vi "XBox Controller.vi"() -> ()   [LabVIEW 2015]
uses:
  XBox-Button States.ctl
  Microsoft.Xna.Framework
  XBox-Globals.vi
panel:
  out "Connected?":bool
  out "Mouse Wheel":i32
  out "Right Trigger":dbl(slide) scale=0.0..1.0
  out "Left Trigger":dbl(slide) scale=0.0..1.0
  out "LeftX":dbl(slide) scale=-1.0..1.0
  out "LeftY":dbl(slide) scale=-1.0..1.0
  out "Left Stick":bool
  out "Left":bool
  out "Right":bool
  out "Down":bool
  out "Up":bool
  out "Right Stick":bool
  out "RightX":dbl(slide) scale=-1.0..1.0
  out "RightY":dbl(slide) scale=-1.0..1.0
  out "Back":bool
  out "Start":bool
  out "Big Button":bool
  out "Left":bool
  out "Right":bool
  out "X":bool
  out "A":bool
  out "B":bool
  out "Y":bool
  in  "Quit":bool
  in  "poll interval (ms)":u32=100
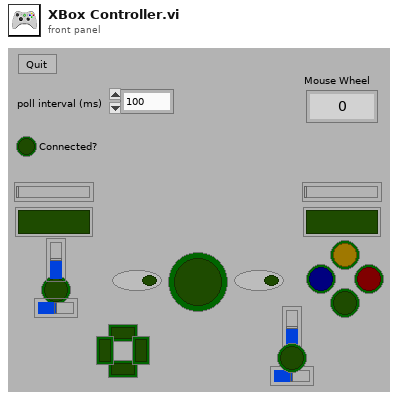
[diagram p1: front panel]
types:
  T1 = typedef "XBox-Button States.ctl" = cluster{"A":bool, "B":bool, "X":bool, "Y":bool, "Left":bool, "Right":bool, "Left Stick":bool, "Right Stick":bool, "Back":bool, "Start":bool, "DPad Down":bool, "DPad Up":bool, "DPad Left":bool, "DPad Right":bool}
  T2 = cluster{"Connected":refnum<user-event>, "A Button":refnum<user-event>, "B Button":refnum<user-event>, "X Button":refnum<user-event>, "Y Button":refnum<user-event>, "Left Button":refnum<user-event>, "Right Button":refnum<user-event>, "Left X":refnum<user-event>, "Left Y":refnum<user-event>, "Right X":refnum<user-event>, "Right Y":refnum<user-event>, "Right Trigger":refnum<user-event>, "Right Trigger":refnum<user-event>, "DPad Left":refnum<user-event>, "DPad Right":refnum<user-event>, "DPad Up":refnum<user-event>, "DPad Down":refnum<user-event>, "Mouse Wheel":refnum<user-event>, "Left Stick":refnum<user-event>, "Right Stick":refnum<user-event>, "Back":refnum<user-event>, "Start":refnum<user-event>, "Left XY":refnum<user-event>}
  T3 = typedef "XBox-Events Ref.ctl" = refnum<event-registration>
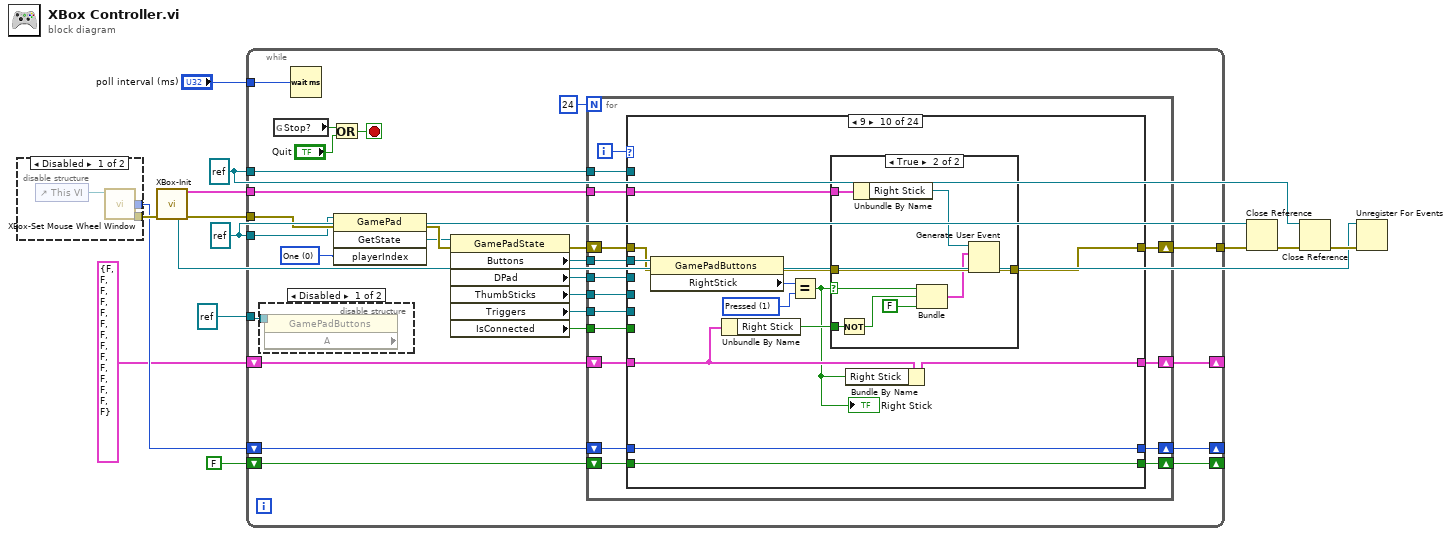
[diagram p0: block diagram]
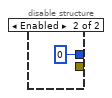
[diagram p2: hidden frame]
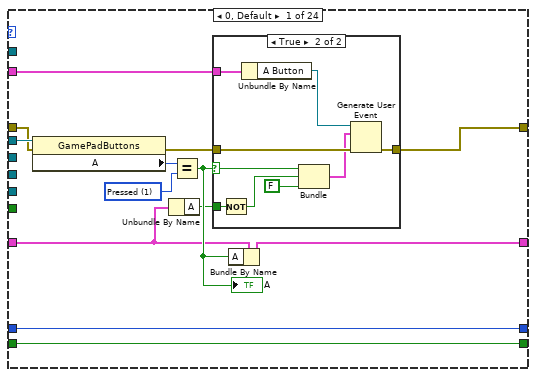
[diagram p4: hidden frame]
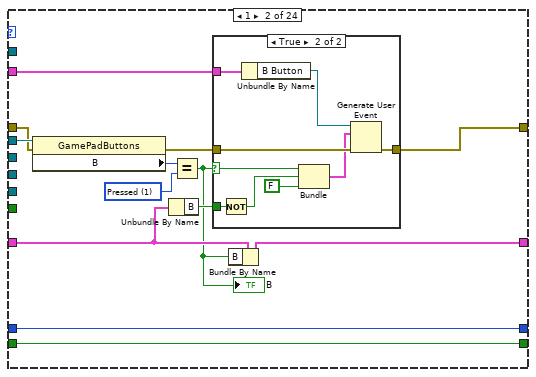
[diagram p6: hidden frame]
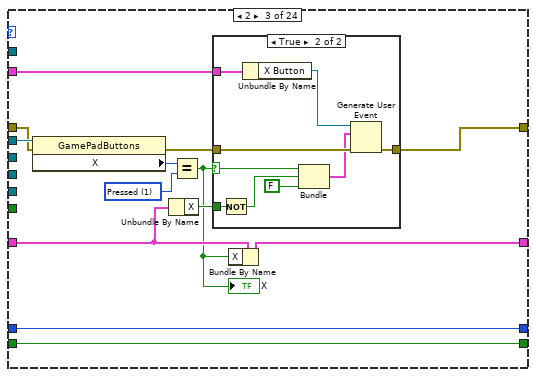
[diagram p8: hidden frame]
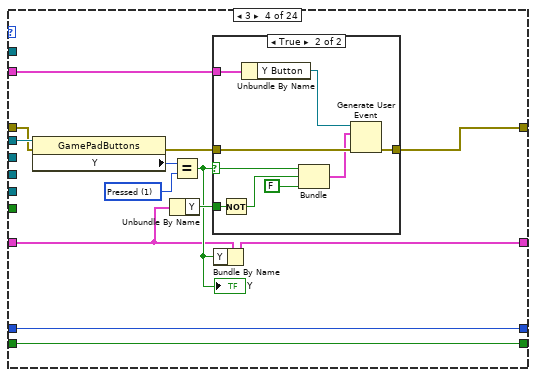
[diagram p10: hidden frame]
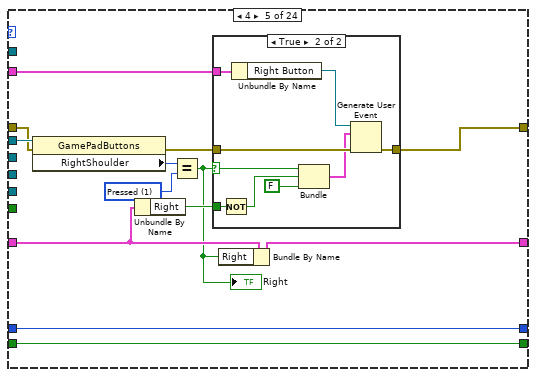
[diagram p12: hidden frame]
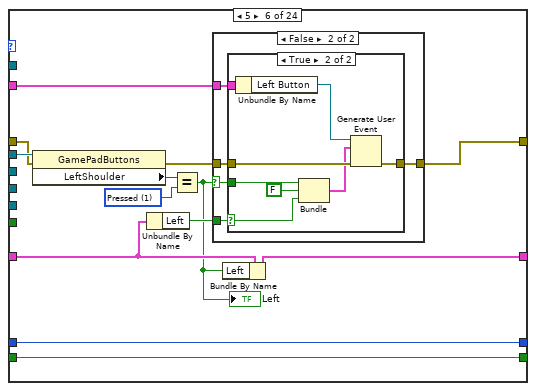
[diagram p14: hidden frame]
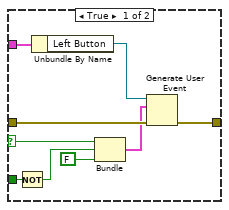
[diagram p15: hidden frame]
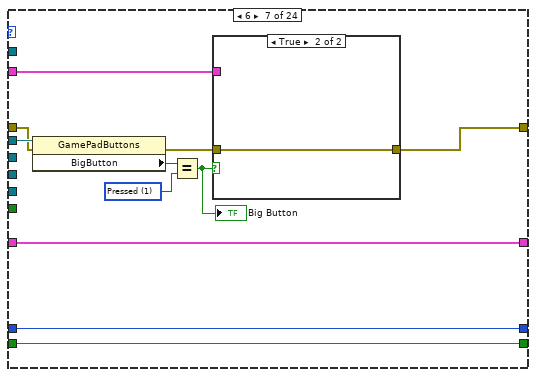
[diagram p17: hidden frame]
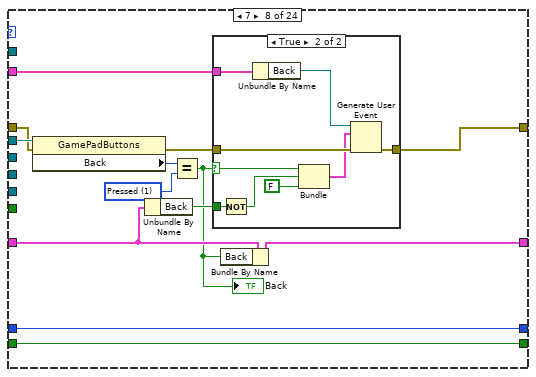
[diagram p19: hidden frame]
diagram:
  w5 = refnum<k24> refnum ("reference")
  w7 = refnum<k24> refnum ("reference")
  n1 = disable-structure shown="Disabled" {
    disable-tunnel: [w16 _] -> w11
    disable-tunnel: [w15 0 ("ScrollWheelValue")] -> w10
    frame Disabled {
      n2 = control-ref of="This VI"() -> (w17:refnum<vi>)
      n3 = call "XBox-Set Mouse Wheel Window.vi"("VI ref"=w17) -> ("ScrollWheelValue"=w15:i32, "error out"=w16:errorcluster)  [unwired: 13 in]
    }
    frame Enabled {
    }
  }
  n4 = call "XBox-Init.vi"("error in (no error)"=w11) -> ("XBox Events"=w12:T2, "Events Ref"=w3:T3, "error out"=w13:errorcluster)  [unwired: 12 in]
  n5 = while {
    tunnel: w12 -> [w39]
    tunnel: "poll interval (ms)" -> [w44]
    tunnel: w13 -> [w38]
    shift-right: [w28] -> _
    shift-left: w10 -> [w29]
    shift-right: [w26] -> _
    shift-left: FALSE -> [w27]
    tunnel: w7 -> [w20]
    tunnel: [w25] -> w8
    tunnel: w5 -> [w24]
    shift-right: [w22] -> _
    shift-left: T1 {"A"=FALSE, "B"=FALSE, "X"=FALSE, "Y"=FALSE, "Left"=FALSE, "Right"=FALSE, "Left Stick"=FALSE, "Right Stick"=FALSE, "Back"=FALSE, "Start"=FALSE, "DPad Down"=FALSE, "DPad Up"=FALSE, "DPad Left"=FALSE, "DPad Right"=FALSE} ("Button States") -> [w23]
    tunnel: refnum<k24> refnum ("reference") -> [w21]
    stop <- w37 stop-if-true
    w43 = 0 items=["One", "Two", "Three", "Four"] ("playerIndex")
    n6 = disable-structure shown="Disabled" {
      disable-tunnel: w21 -> [w45 _]
      frame Disabled {
        n7 = property class="GamePadButtons" props=["A"](reference=w45) -> ()  [unwired: 1 in, 3 out]
      }
      frame Enabled {
      }
    }
    n8 = global read "XBox-Globals.vi" "Stop?"() -> (w36:bool)
    n9 = Wait (ms)(milliseconds to wait=w44) -> ()  [unwired: 1 out]
    n10 = Or(x=w36, y="Quit") -> (x .or. y?=w37:bool)
    n11 = invoke class="GamePad" method="GetState"(reference=w20, error in=w38, "playerIndex"=w43) -> (error out=w42:errorcluster, "GetState"=w19:refnum<k24>)  [unwired: 1 in, 2 out]
    n12 = property class="GamePadState"(reference=w19, error in=w42) -> (error out=w40:errorcluster, "Buttons"=w41:refnum<k24>, "DPad"=w33:refnum<k24>, "ThumbSticks"=w32:refnum<k24>, "Triggers"=w31:refnum<k24>, "IsConnected"=w30:bool)  [unwired: 1 out]
    n13 = for {
      N: 24 -> [_]
      tunnel: w41 -> [w61]
      tunnel: w39 -> [w59]
      shift-right: [w57] -> w25
      shift-left: w40 -> [w60]
      tunnel: w33 -> [w56]
      tunnel: w32 -> [w55]
      tunnel: w31 -> [w54]
      tunnel: w30 -> [w53]
      shift-right: [w51] -> w28
      shift-left: w29 -> [w52]
      shift-right: [w49] -> w26
      shift-left: w27 -> [w50]
      tunnel: w24 -> [w48]
      shift-right: [w46] -> w22
      shift-left: w23 -> [w47]
      i -> [w58]
      n14 = case shown="9" w58 {
        tunnel: w61 -> [w74 w97 w120 w143 w166 w189 w223 w238 w261 w284 w307 _ _ _ _ _ _ _ _ _ _ _ _ _]
        tunnel: w60 -> [w69 w92 w115 w138 w161 w184 w218 w233 w256 w279 w302 w318 w342 w365 w388 w421 w440 w459 w478 w495 w512 _ w541 w558]
        tunnel: w59 -> [w71 w94 w117 w140 w163 w186 w220 w235 w258 w281 w304 w328 w351 w374 w397 w422 w441 w460 w479 w496 w513 w527 w542 w560]
        tunnel: [w68 w91 w114 w137 w160 w183 w217 w232 w255 w278 w301 w326 w349 w372 w395 w420 w439 w458 w477 w494 w511 w525 w539 w557] -> w57
        tunnel: w56 -> [_ _ _ _ _ _ _ _ _ _ _ w319 w343 w366 w389 _ _ _ _ _ _ _ _ _]
        tunnel: w55 -> [_ _ _ _ _ _ _ _ _ _ _ _ _ _ _ w419 w438 w457 w476 _ _ _ _ w559]
        tunnel: w54 -> [_ _ _ _ _ _ _ _ _ _ _ _ _ _ _ _ _ _ _ w491 w508 _ _ _]
        tunnel: w53 -> [_ _ _ _ _ _ _ _ _ _ _ _ _ _ _ _ _ _ _ _ _ _ w536 _]
        tunnel: w52 -> [w67 w90 w113 w136 w159 w182 w215 w231 w254 w277 w300 w325 w348 w371 w394 w412 w431 w450 w469 w488 w505 w529 w538 w555]
        tunnel: [w67 w90 w113 w136 w159 w182 w215 w231 w254 w277 w300 w325 w348 w371 w394 w412 w431 w450 w469 w488 w505 w521 w538 w555] -> w51
        tunnel: w50 -> [w66 w89 w112 w135 w158 w181 w214 w230 w253 w276 w299 w324 w347 w370 w393 w411 w430 w449 w468 w487 w504 w528 w543 w554]
        tunnel: [w66 w89 w112 w135 w158 w181 w214 w230 w253 w276 w299 w324 w347 w370 w393 w411 w430 w449 w468 w487 w504 w528 w536 w554] -> w49
        tunnel: w48 -> [_ _ _ _ _ _ _ _ _ _ _ _ _ _ _ _ _ _ _ _ _ w520 _ _]
        tunnel: w47 -> [w63 w87 w110 w131 w156 w179 w213 w228 w251 w274 w297 w322 w345 w368 w391 w410 w429 w448 w467 w486 w503 w524 w537 w556]
        tunnel: [w64 w88 w111 w134 w157 w180 w213 w229 w252 w275 w298 w323 w346 w369 w392 w410 w429 w448 w467 w486 w503 w524 w537 w556] -> w46
        frame 0, Default {
          w73 = 1 items=["Released", "Pressed"] ("Y")
          n15 = property class="GamePadButtons"(reference=w74, error in=w69) -> (error out=w70:errorcluster, "A"=w72:i32)  [unwired: 1 out]
          n16 = Unbundle By Name(w63) -> ("A"=w62:bool)
          n17 = Equal?(x=w72, y=w73) -> (x = y?=w65:bool)
          "A" <- w65
          n18 = case shown="True" w65 {
            selector: w65 -> [_ w80]
            tunnel: w71 -> [_ w84]
            tunnel: w70 -> [w75 w83]
            tunnel: [w75 w81] -> w68
            tunnel: w62 -> [_ w79]
            frame False {
            }
            frame True {
              n19 = Not(x=w79) -> (.not. x?=w76:bool)
              n20 = Unbundle By Name(w84) -> ("A Button"=w82:refnum<user-event>)
              n21 = Bundle(w80, w76, FALSE) -> (w77:cluster{bool, bool, bool})  [unwired: 1 in]
              n22 = Generate User Event(user event=w82, event data cluster=w77, error in=w83) -> (error out=w81:errorcluster)  [unwired: 1 in, 1 out]
            }
          }
          n23 = Bundle By Name(cluster=w63, "A"=w65) -> (w64:T1)
        }
        frame 1 {
          w96 = 1 items=["Released", "Pressed"] ("Y")
          n24 = property class="GamePadButtons"(reference=w97, error in=w92) -> (error out=w93:errorcluster, "B"=w95:i32)  [unwired: 1 out]
          n25 = Unbundle By Name(w87) -> ("B"=w86:bool)
          n26 = Equal?(x=w95, y=w96) -> (x = y?=w85:bool)
          "B" <- w85
          n27 = case shown="True" w85 {
            selector: w85 -> [_ w103]
            tunnel: w94 -> [_ w107]
            tunnel: w93 -> [w98 w106]
            tunnel: [w98 w104] -> w91
            tunnel: w86 -> [_ w102]
            frame False {
            }
            frame True {
              n28 = Not(x=w102) -> (.not. x?=w99:bool)
              n29 = Unbundle By Name(w107) -> ("B Button"=w105:refnum<user-event>)
              n30 = Bundle(w103, w99, FALSE) -> (w100:cluster{bool, bool, bool})  [unwired: 1 in]
              n31 = Generate User Event(user event=w105, event data cluster=w100, error in=w106) -> (error out=w104:errorcluster)  [unwired: 1 in, 1 out]
            }
          }
          n32 = Bundle By Name(cluster=w87, "B"=w85) -> (w88:T1)
        }
        frame 2 {
          w119 = 1 items=["Released", "Pressed"] ("Y")
          n33 = property class="GamePadButtons"(reference=w120, error in=w115) -> (error out=w116:errorcluster, "X"=w118:i32)  [unwired: 1 out]
          n34 = Unbundle By Name(w110) -> ("X"=w109:bool)
          n35 = Equal?(x=w118, y=w119) -> (x = y?=w108:bool)
          "X" <- w108
          n36 = case shown="True" w108 {
            selector: w108 -> [_ w126]
            tunnel: w117 -> [_ w130]
            tunnel: w116 -> [w121 w129]
            tunnel: [w121 w127] -> w114
            tunnel: w109 -> [_ w125]
            frame False {
            }
            frame True {
              n37 = Not(x=w125) -> (.not. x?=w122:bool)
              n38 = Unbundle By Name(w130) -> ("X Button"=w128:refnum<user-event>)
              n39 = Bundle(w126, w122, FALSE) -> (w123:cluster{bool, bool, bool})  [unwired: 1 in]
              n40 = Generate User Event(user event=w128, event data cluster=w123, error in=w129) -> (error out=w127:errorcluster)  [unwired: 1 in, 1 out]
            }
          }
          n41 = Bundle By Name(cluster=w110, "X"=w108) -> (w111:T1)
        }
        frame 3 {
          w142 = 1 items=["Released", "Pressed"] ("Y")
          n42 = property class="GamePadButtons"(reference=w143, error in=w138) -> (error out=w139:errorcluster, "Y"=w141:i32)  [unwired: 1 out]
          n43 = Unbundle By Name(w131) -> ("Y"=w133:bool)
          n44 = Equal?(x=w141, y=w142) -> (x = y?=w132:bool)
          "Y" <- w132
          n45 = case shown="True" w132 {
            selector: w132 -> [_ w149]
            tunnel: w140 -> [_ w153]
            tunnel: w139 -> [w144 w152]
            tunnel: [w144 w150] -> w137
            tunnel: w133 -> [_ w148]
            frame False {
            }
            frame True {
              n46 = Not(x=w148) -> (.not. x?=w145:bool)
              n47 = Unbundle By Name(w153) -> ("Y Button"=w151:refnum<user-event>)
              n48 = Bundle(w149, w145, FALSE) -> (w146:cluster{bool, bool, bool})  [unwired: 1 in]
              n49 = Generate User Event(user event=w151, event data cluster=w146, error in=w152) -> (error out=w150:errorcluster)  [unwired: 1 in, 1 out]
            }
          }
          n50 = Bundle By Name(cluster=w131, "Y"=w132) -> (w134:T1)
        }
        frame 4 {
          w165 = 1 items=["Released", "Pressed"] ("Y")
          n51 = property class="GamePadButtons"(reference=w166, error in=w161) -> (error out=w162:errorcluster, "RightShoulder"=w164:i32)  [unwired: 1 out]
          n52 = Unbundle By Name(w156) -> ("Right"=w155:bool)
          n53 = Equal?(x=w164, y=w165) -> (x = y?=w154:bool)
          "Right" <- w154
          n54 = case shown="True" w154 {
            selector: w154 -> [_ w172]
            tunnel: w163 -> [_ w176]
            tunnel: w162 -> [w167 w175]
            tunnel: [w167 w173] -> w160
            tunnel: w155 -> [_ w171]
            frame False {
            }
            frame True {
              n55 = Not(x=w171) -> (.not. x?=w168:bool)
              n56 = Unbundle By Name(w176) -> ("Right Button"=w174:refnum<user-event>)
              n57 = Bundle(w172, w168, FALSE) -> (w169:cluster{bool, bool, bool})  [unwired: 1 in]
              n58 = Generate User Event(user event=w174, event data cluster=w169, error in=w175) -> (error out=w173:errorcluster)  [unwired: 1 in, 1 out]
            }
          }
          n59 = Bundle By Name(cluster=w156, "Right"=w154) -> (w157:T1)
        }
        frame 5 {
          w188 = 1 items=["Released", "Pressed"] ("Y")
          n60 = property class="GamePadButtons"(reference=w189, error in=w184) -> (error out=w185:errorcluster, "LeftShoulder"=w187:i32)  [unwired: 1 out]
          n61 = Unbundle By Name(w179) -> ("Left"=w178:bool)
          n62 = Equal?(x=w187, y=w188) -> (x = y?=w177:bool)
          "Left" <- w177
          n63 = case shown="False" w177 {
            selector: w177 -> [w194 w200]
            tunnel: w186 -> [w198 w203]
            tunnel: w185 -> [w197 w202]
            tunnel: [w195 w201] -> w183
            tunnel: w178 -> [w193 w199]
            frame True {
              n64 = Not(x=w193) -> (.not. x?=w190:bool)
              n65 = Unbundle By Name(w198) -> ("Left Button"=w196:refnum<user-event>)
              n66 = Bundle(w194, w190, FALSE) -> (w191:cluster{bool, bool, bool})  [unwired: 1 in]
              n67 = Generate User Event(user event=w196, event data cluster=w191, error in=w197) -> (error out=w195:errorcluster)  [unwired: 1 in, 1 out]
            }
            frame False {
              n68 = case shown="True" w199 {
                selector: w199 -> [_ w205]
                tunnel: w203 -> [_ w212]
                tunnel: w202 -> [w204 w211]
                tunnel: [w204 w209] -> w201
                tunnel: w200 -> [_ w208]
                frame False {
                }
                frame True {
                  n69 = Unbundle By Name(w212) -> ("Left Button"=w210:refnum<user-event>)
                  n70 = Bundle(w208, FALSE, w205) -> (w207:cluster{bool, bool, bool})  [unwired: 1 in]
                  n71 = Generate User Event(user event=w210, event data cluster=w207, error in=w211) -> (error out=w209:errorcluster)  [unwired: 1 in, 1 out]
                }
              }
            }
          }
          n72 = Bundle By Name(cluster=w179, "Left"=w177) -> (w180:T1)
        }
        frame 6 {
          w222 = 1 items=["Released", "Pressed"] ("Y")
          n73 = property class="GamePadButtons"(reference=w223, error in=w218) -> (error out=w219:errorcluster, "BigButton"=w221:i32)  [unwired: 1 out]
          n74 = Equal?(x=w221, y=w222) -> (x = y?=w216:bool)
          "Big Button" <- w216
          n75 = case shown="True" w216 {
            tunnel: w220 -> [_ _]
            tunnel: w219 -> [w224 w225]
            tunnel: [w224 w225] -> w217
            frame False {
            }
            frame True {
            }
          }
        }
        frame 7 {
          w237 = 1 items=["Released", "Pressed"] ("Y")
          n76 = property class="GamePadButtons"(reference=w238, error in=w233) -> (error out=w234:errorcluster, "Back"=w236:i32)  [unwired: 1 out]
          n77 = Unbundle By Name(w228) -> ("Back"=w227:bool)
          n78 = Equal?(x=w236, y=w237) -> (x = y?=w226:bool)
          "Back" <- w226
          n79 = case shown="True" w226 {
            selector: w226 -> [_ w244]
            tunnel: w235 -> [_ w248]
            tunnel: w234 -> [w239 w247]
            tunnel: [w239 w245] -> w232
            tunnel: w227 -> [_ w243]
            frame False {
            }
            frame True {
              n80 = Not(x=w243) -> (.not. x?=w240:bool)
              n81 = Unbundle By Name(w248) -> ("Back"=w246:refnum<user-event>)
              n82 = Bundle(w244, w240, FALSE) -> (w241:cluster{bool, bool, bool})  [unwired: 1 in]
              n83 = Generate User Event(user event=w246, event data cluster=w241, error in=w247) -> (error out=w245:errorcluster)  [unwired: 1 in, 1 out]
            }
          }
          n84 = Bundle By Name(cluster=w228, "Back"=w226) -> (w229:T1)
        }
        frame 8 {
          w260 = 1 items=["Released", "Pressed"] ("Y")
          n85 = property class="GamePadButtons"(reference=w261, error in=w256) -> (error out=w257:errorcluster, "Start"=w259:i32)  [unwired: 1 out]
          n86 = Unbundle By Name(w251) -> ("Start"=w250:bool)
          n87 = Equal?(x=w259, y=w260) -> (x = y?=w249:bool)
          "Start" <- w249
          n88 = case shown="True" w249 {
            selector: w249 -> [_ w267]
            tunnel: w258 -> [_ w271]
            tunnel: w257 -> [w262 w270]
            tunnel: [w262 w268] -> w255
            tunnel: w250 -> [_ w266]
            frame False {
            }
            frame True {
              n89 = Not(x=w266) -> (.not. x?=w263:bool)
              n90 = Unbundle By Name(w271) -> ("Start"=w269:refnum<user-event>)
              n91 = Bundle(w267, w263, FALSE) -> (w264:cluster{bool, bool, bool})  [unwired: 1 in]
              n92 = Generate User Event(user event=w269, event data cluster=w264, error in=w270) -> (error out=w268:errorcluster)  [unwired: 1 in, 1 out]
            }
          }
          n93 = Bundle By Name(cluster=w251, "Start"=w249) -> (w252:T1)
        }
        frame 9 {
          w283 = 1 items=["Released", "Pressed"] ("Y")
          n94 = property class="GamePadButtons"(reference=w284, error in=w279) -> (error out=w280:errorcluster, "RightStick"=w282:i32)  [unwired: 1 out]
          n95 = Unbundle By Name(w274) -> ("Right Stick"=w273:bool)
          n96 = Equal?(x=w282, y=w283) -> (x = y?=w272:bool)
          "Right Stick" <- w272
          n97 = case shown="True" w272 {
            selector: w272 -> [_ w290]
            tunnel: w281 -> [_ w294]
            tunnel: w280 -> [w285 w293]
            tunnel: [w285 w291] -> w278
            tunnel: w273 -> [_ w289]
            frame False {
            }
            frame True {
              n98 = Not(x=w289) -> (.not. x?=w286:bool)
              n99 = Unbundle By Name(w294) -> ("Right Stick"=w292:refnum<user-event>)
              n100 = Bundle(w290, w286, FALSE) -> (w287:cluster{bool, bool, bool})  [unwired: 1 in]
              n101 = Generate User Event(user event=w292, event data cluster=w287, error in=w293) -> (error out=w291:errorcluster)  [unwired: 1 in, 1 out]
            }
          }
          n102 = Bundle By Name(cluster=w274, "Right Stick"=w272) -> (w275:T1)
        }
        frame 10 {
          w306 = 1 items=["Released", "Pressed"] ("Y")
          n103 = property class="GamePadButtons"(reference=w307, error in=w302) -> (error out=w303:errorcluster, "LeftStick"=w305:i32)  [unwired: 1 out]
          n104 = Unbundle By Name(w297) -> ("Left Stick"=w296:bool)
          n105 = Equal?(x=w305, y=w306) -> (x = y?=w295:bool)
          "Left Stick" <- w295
          n106 = Bundle By Name(cluster=w297, "Left Stick"=w295) -> (w298:T1)
          n107 = case shown="True" w295 {
            selector: w295 -> [_ w313]
            tunnel: w304 -> [_ w317]
            tunnel: w303 -> [w308 w316]
            tunnel: [w308 w314] -> w301
            tunnel: w296 -> [_ w312]
            frame False {
            }
            frame True {
              n108 = Not(x=w312) -> (.not. x?=w309:bool)
              n109 = Unbundle By Name(w317) -> ("Left Stick"=w315:refnum<user-event>)
              n110 = Bundle(w313, w309, FALSE) -> (w310:cluster{bool, bool, bool})  [unwired: 1 in]
              n111 = Generate User Event(user event=w315, event data cluster=w310, error in=w316) -> (error out=w314:errorcluster)  [unwired: 1 in, 1 out]
            }
          }
        }
        frame 11 {
          w330 = 1 items=["Released", "Pressed"] ("Y")
          n112 = property class="GamePadDPad"(reference=w319, error in=w318) -> (error out=w327:errorcluster, "Down"=w329:i32)  [unwired: 1 out]
          n113 = Unbundle By Name(w322) -> ("DPad Down"=w321:bool)
          n114 = Equal?(x=w329, y=w330) -> (x = y?=w320:bool)
          "Down" <- w320
          n115 = case shown="True" w320 {
            selector: w320 -> [_ w336]
            tunnel: w328 -> [_ w340]
            tunnel: w327 -> [w331 w339]
            tunnel: [w331 w337] -> w326
            tunnel: w321 -> [_ w335]
            frame False {
            }
            frame True {
              n116 = Not(x=w335) -> (.not. x?=w332:bool)
              n117 = Unbundle By Name(w340) -> ("DPad Down"=w338:refnum<user-event>)
              n118 = Bundle(w336, w332, FALSE) -> (w333:cluster{bool, bool, bool})  [unwired: 1 in]
              n119 = Generate User Event(user event=w338, event data cluster=w333, error in=w339) -> (error out=w337:errorcluster)  [unwired: 1 in, 1 out]
            }
          }
          n120 = Bundle By Name(cluster=w322, "DPad Down"=w320) -> (w323:T1)
        }
        frame 12 {
          w353 = 1 items=["Released", "Pressed"] ("Y")
          n121 = property class="GamePadDPad"(reference=w343, error in=w342) -> (error out=w350:errorcluster, "Up"=w352:i32)  [unwired: 1 out]
          n122 = Unbundle By Name(w345) -> ("DPad Up"=w344:bool)
          n123 = Equal?(x=w352, y=w353) -> (x = y?=w341:bool)
          "Up" <- w341
          n124 = case shown="True" w341 {
            selector: w341 -> [_ w359]
            tunnel: w351 -> [_ w363]
            tunnel: w350 -> [w354 w362]
            tunnel: [w354 w360] -> w349
            tunnel: w344 -> [_ w358]
            frame False {
            }
            frame True {
              n125 = Not(x=w358) -> (.not. x?=w355:bool)
              n126 = Unbundle By Name(w363) -> ("DPad Up"=w361:refnum<user-event>)
              n127 = Bundle(w359, w355, FALSE) -> (w356:cluster{bool, bool, bool})  [unwired: 1 in]
              n128 = Generate User Event(user event=w361, event data cluster=w356, error in=w362) -> (error out=w360:errorcluster)  [unwired: 1 in, 1 out]
            }
          }
          n129 = Bundle By Name(cluster=w345, "DPad Up"=w341) -> (w346:T1)
        }
        frame 13 {
          w376 = 1 items=["Released", "Pressed"] ("Y")
          n130 = property class="GamePadDPad"(reference=w366, error in=w365) -> (error out=w373:errorcluster, "Left"=w375:i32)  [unwired: 1 out]
          n131 = Unbundle By Name(w368) -> ("DPad Left"=w367:bool)
          n132 = Equal?(x=w375, y=w376) -> (x = y?=w364:bool)
          "Left" <- w364
          n133 = case shown="True" w364 {
            selector: w364 -> [_ w382]
            tunnel: w374 -> [_ w386]
            tunnel: w373 -> [w377 w385]
            tunnel: [w377 w383] -> w372
            tunnel: w367 -> [_ w381]
            frame False {
            }
            frame True {
              n134 = Not(x=w381) -> (.not. x?=w378:bool)
              n135 = Unbundle By Name(w386) -> ("DPad Left"=w384:refnum<user-event>)
              n136 = Bundle(w382, w378, FALSE) -> (w379:cluster{bool, bool, bool})  [unwired: 1 in]
              n137 = Generate User Event(user event=w384, event data cluster=w379, error in=w385) -> (error out=w383:errorcluster)  [unwired: 1 in, 1 out]
            }
          }
          n138 = Bundle By Name(cluster=w368, "DPad Left"=w364) -> (w369:T1)
        }
        frame 14 {
          w399 = 1 items=["Released", "Pressed"] ("Y")
          n139 = property class="GamePadDPad"(reference=w389, error in=w388) -> (error out=w396:errorcluster, "Right"=w398:i32)  [unwired: 1 out]
          n140 = Unbundle By Name(w391) -> ("DPad Right"=w390:bool)
          n141 = Equal?(x=w398, y=w399) -> (x = y?=w387:bool)
          "Right" <- w387
          n142 = case shown="True" w387 {
            selector: w387 -> [_ w405]
            tunnel: w397 -> [_ w409]
            tunnel: w396 -> [w400 w408]
            tunnel: [w400 w406] -> w395
            tunnel: w390 -> [_ w404]
            frame False {
            }
            frame True {
              n143 = Not(x=w404) -> (.not. x?=w401:bool)
              n144 = Unbundle By Name(w409) -> ("DPad Right"=w407:refnum<user-event>)
              n145 = Bundle(w405, w401, FALSE) -> (w402:cluster{bool, bool, bool})  [unwired: 1 in]
              n146 = Generate User Event(user event=w407, event data cluster=w402, error in=w408) -> (error out=w406:errorcluster)  [unwired: 1 in, 1 out]
            }
          }
          n147 = Bundle By Name(cluster=w391, "DPad Right"=w387) -> (w392:T1)
        }
        frame 15 {
          n148 = property class="GamePadThumbSticks"(reference=w419, error in=w421) -> (error out=w417:errorcluster, "Right"=w418:refnum<k24>)  [unwired: 1 out]
          n149 = property class="Vector2"(reference=w418, error in=w417) -> (error out=w416:errorcluster, "Y"=w413:sgl)  [unwired: 1 out]
          "RightY" <- w413
          n150 = Absolute Value(x=w413) -> (abs(x)=w415:sgl)
          n151 = Greater Than 0?(x=w415) -> (x > 0?=w414:bool)
          n152 = case shown="True" w414 {
            tunnel: w422 -> [_ w428]
            tunnel: w416 -> [w423 w426]
            tunnel: [w423 w427] -> w420
            tunnel: w413 -> [_ w424]
            frame False {
            }
            frame True {
              n153 = Unbundle By Name(w428) -> ("Right Y"=w425:refnum<user-event>)
              n154 = Generate User Event(user event=w425, event data cluster=w424, error in=w426) -> (error out=w427:errorcluster)  [unwired: 1 in, 1 out]
            }
          }
        }
        frame 16 {
          n155 = property class="GamePadThumbSticks"(reference=w438, error in=w440) -> (error out=w436:errorcluster, "Right"=w437:refnum<k24>)  [unwired: 1 out]
          n156 = property class="Vector2"(reference=w437, error in=w436) -> (error out=w435:errorcluster, "X"=w432:sgl)  [unwired: 1 out]
          "RightX" <- w432
          n157 = Absolute Value(x=w432) -> (abs(x)=w434:sgl)
          n158 = Greater Than 0?(x=w434) -> (x > 0?=w433:bool)
          n159 = case shown="True" w433 {
            tunnel: w441 -> [_ w447]
            tunnel: w435 -> [w442 w445]
            tunnel: [w442 w446] -> w439
            tunnel: w432 -> [_ w443]
            frame False {
            }
            frame True {
              n160 = Unbundle By Name(w447) -> ("Right X"=w444:refnum<user-event>)
              n161 = Generate User Event(user event=w444, event data cluster=w443, error in=w445) -> (error out=w446:errorcluster)  [unwired: 1 in, 1 out]
            }
          }
        }
        frame 17 {
          n162 = property class="GamePadThumbSticks"(reference=w457, error in=w459) -> (error out=w455:errorcluster, "Left"=w456:refnum<k24>)  [unwired: 1 out]
          n163 = property class="Vector2"(reference=w456, error in=w455) -> (error out=w454:errorcluster, "Y"=w451:sgl)  [unwired: 1 out]
          "LeftY" <- w451
          n164 = Absolute Value(x=w451) -> (abs(x)=w453:sgl)
          n165 = Greater Than 0?(x=w453) -> (x > 0?=w452:bool)
          n166 = case shown="True" w452 {
            tunnel: w460 -> [_ w466]
            tunnel: w454 -> [w461 w464]
            tunnel: [w461 w465] -> w458
            tunnel: w451 -> [_ w462]
            frame False {
            }
            frame True {
              n167 = Unbundle By Name(w466) -> ("Left Y"=w463:refnum<user-event>)
              n168 = Generate User Event(user event=w463, event data cluster=w462, error in=w464) -> (error out=w465:errorcluster)  [unwired: 1 in, 1 out]
            }
          }
        }
        frame 18 {
          n169 = property class="GamePadThumbSticks"(reference=w476, error in=w478) -> (error out=w474:errorcluster, "Left"=w475:refnum<k24>)  [unwired: 1 out]
          n170 = property class="Vector2"(reference=w475, error in=w474) -> (error out=w473:errorcluster, "X"=w470:sgl)  [unwired: 1 out]
          "LeftX" <- w470
          n171 = Absolute Value(x=w470) -> (abs(x)=w472:sgl)
          n172 = Greater Than 0?(x=w472) -> (x > 0?=w471:bool)
          n173 = case shown="True" w471 {
            tunnel: w479 -> [_ w485]
            tunnel: w473 -> [w480 w483]
            tunnel: [w480 w484] -> w477
            tunnel: w470 -> [_ w481]
            frame False {
            }
            frame True {
              n174 = Unbundle By Name(w485) -> ("Left X"=w482:refnum<user-event>)
              n175 = Generate User Event(user event=w482, event data cluster=w481, error in=w483) -> (error out=w484:errorcluster)  [unwired: 1 in, 1 out]
            }
          }
        }
        frame 19 {
          n176 = property class="GamePadTriggers"(reference=w491, error in=w495) -> (error out=w489:errorcluster, "Left"=w490:sgl)  [unwired: 1 out]
          "Left Trigger" <- w490
          n177 = Absolute Value(x=w490) -> (abs(x)=w493:sgl)
          n178 = Greater Than 0?(x=w493) -> (x > 0?=w492:bool)
          n179 = case shown="True" w492 {
            tunnel: w496 -> [_ w502]
            tunnel: w489 -> [w497 w500]
            tunnel: [w497 w501] -> w494
            tunnel: w490 -> [_ w498]
            frame False {
            }
            frame True {
              n180 = Unbundle By Name(w502) -> ("Right Trigger"=w499:refnum<user-event>)
              n181 = Generate User Event(user event=w499, event data cluster=w498, error in=w500) -> (error out=w501:errorcluster)  [unwired: 1 in, 1 out]
            }
          }
        }
        frame 20 {
          n182 = property class="GamePadTriggers"(reference=w508, error in=w512) -> (error out=w507:errorcluster, "Right"=w506:sgl)  [unwired: 1 out]
          "Right Trigger" <- w506
          n183 = Absolute Value(x=w506) -> (abs(x)=w510:sgl)
          n184 = Greater Than 0?(x=w510) -> (x > 0?=w509:bool)
          n185 = case shown="True" w509 {
            tunnel: w513 -> [_ w519]
            tunnel: w507 -> [w514 w517]
            tunnel: [w514 w518] -> w511
            tunnel: w506 -> [_ w515]
            frame False {
            }
            frame True {
              n186 = Unbundle By Name(w519) -> ("Right Trigger"=w516:refnum<user-event>)
              n187 = Generate User Event(user event=w516, event data cluster=w515, error in=w517) -> (error out=w518:errorcluster)  [unwired: 1 in, 1 out]
            }
          }
        }
        frame 21 {
          n188 = property class="MouseState"(reference=w520) -> (error out=w522:errorcluster, "ScrollWheelValue"=w521:i32)  [unwired: 1 in, 1 out]
          n189 = Subtract(x=w521, y=w529) -> (x-y=w526:i32)
          "Mouse Wheel" <- w526
          n190 = Not Equal To 0?(x=w526) -> (x != 0?=w523:bool)
          n191 = case shown="True" w523 {
            tunnel: w522 -> [w530 w535]
            tunnel: w527 -> [_ w534]
            tunnel: w526 -> [_ w532]
            tunnel: [w530 w531] -> w525
            frame False {
            }
            frame True {
              n192 = Unbundle By Name(w534) -> ("Mouse Wheel"=w533:refnum<user-event>)
              n193 = Generate User Event(user event=w533, event data cluster=w532, error in=w535) -> (error out=w531:errorcluster)  [unwired: 1 in, 1 out]
            }
          }
        }
        frame 22 {
          n194 = Not Equal?(x=w536, y=w543) -> (x != y?=w540:bool)
          n195 = global write "XBox-Globals.vi" "Connected?"(w536) -> ()
          n196 = case shown="True" w540 {
            tunnel: w542 -> [_ w549]
            tunnel: w541 -> [w544 w548]
            tunnel: w536 -> [_ w546]
            tunnel: [w544 w545] -> w539
            frame False {
            }
            frame True {
              n197 = Unbundle By Name(w549) -> ("Connected"=w547:refnum<user-event>)
              n198 = Generate User Event(user event=w547, event data cluster=w546, error in=w548) -> (error out=w545:errorcluster)  [unwired: 1 in, 1 out]
            }
          }
          "Connected?" <- w536
        }
        frame 23 {
          n199 = property class="GamePadThumbSticks"(reference=w559, error in=w558) -> (error out=w562:errorcluster, "Left"=w561:refnum<k24>)  [unwired: 1 out]
          n200 = property class="Vector2"(reference=w561, error in=w562) -> (error out=w563:errorcluster, "X"=w566:sgl, "Y"=w552:sgl)  [unwired: 1 out]
          n201 = Absolute Value(x=w566) -> (abs(x)=w564:sgl)
          n202 = Absolute Value(x=w552) -> (abs(x)=w553:sgl)
          n203 = Greater Than 0?(x=w564) -> (x > 0?=w565:bool)
          n204 = Greater Than 0?(x=w553) -> (x > 0?=w550:bool)
          n205 = Or(x=w565, y=w550) -> (x .or. y?=w551:bool)
          n206 = case shown="True" w551 {
            tunnel: w560 -> [_ w574]
            tunnel: w563 -> [w567 w572]
            tunnel: [w567 w573] -> w557
            tunnel: w566 -> [_ w570]
            tunnel: w552 -> [_ w569]
            frame False {
            }
            frame True {
              n207 = Unbundle By Name(w574) -> ("Left XY"=w571:refnum<user-event>)
              n208 = Bundle("X"=w570, "Y"=w569) -> (w568:cluster{"X":sgl, "Y":sgl})  [unwired: 1 in]
              n209 = Generate User Event(user event=w571, event data cluster=w568, error in=w572) -> (error out=w573:errorcluster)  [unwired: 1 in, 1 out]
            }
          }
        }
      }
    }
  }
  n210 = Close Reference(reference=w7, error in (no error)=w8) -> (error out=w6:errorcluster)
  n211 = Close Reference(reference=w5, error in (no error)=w6) -> (error out=w4:errorcluster)
  n212 = Unregister For Events(event registration refnum=w3, error in=w4) -> ()  [unwired: 1 out]
